vi "alloc_and_project_patterns_dmd.vi"(8 "Path":path, 9 "PicNum":i32, 10 "load patterns":bool, 11 "PictureTime":i32) -> (0 "return array":i32[](array[numeric]), 1 "SeqId":u32, 2 "DevId":u32)   [LabVIEW 2019]
uses:
  <userlib>/alp4395/alp4395.lvlib
  <userlib>/alp4395/alp4395.dll
panel:
  out "path":path
  out "function return 10":i32
  out "function return 6":i32
  out "function return 9":i32
  out "function return 7":i32
  out "function return 5":i32
  out "function return 4":i32
  out "array":u8[][][](array[numeric])
  out "function return 3":i32
  out "function return 2":i32
  out "function return 8":i32
  out "function return":i32
  out "height":i32
  out "width":i32
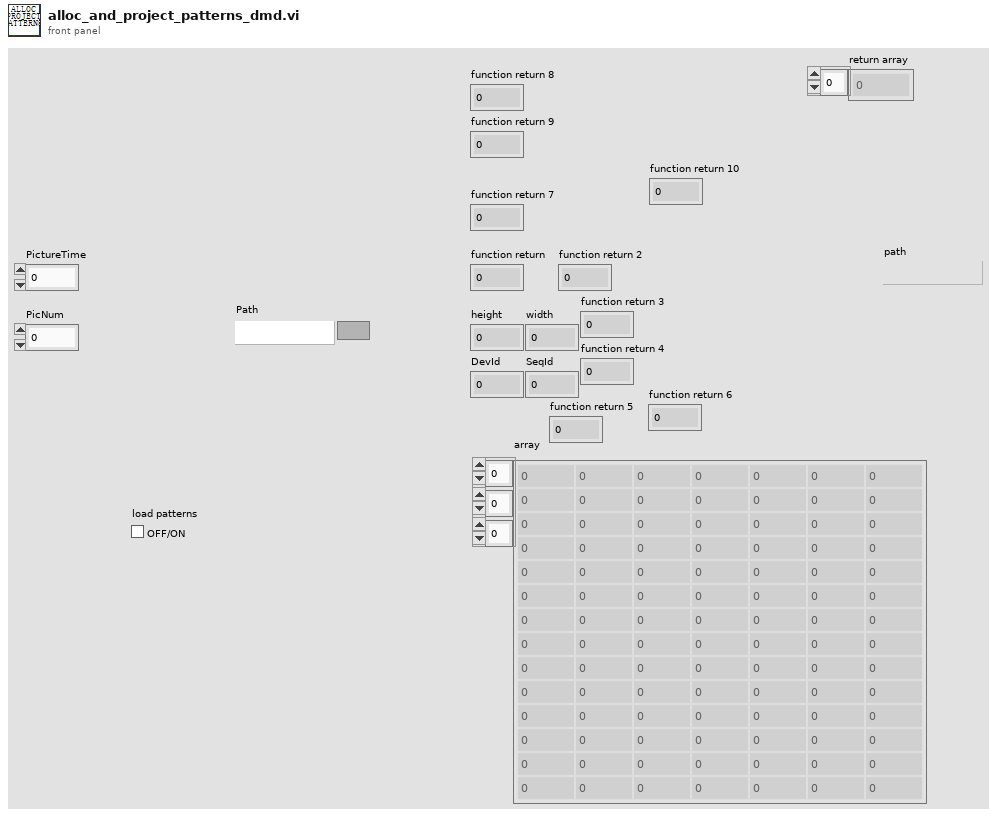
[diagram p1: front panel]
types:
  T1 = typedef "IMAQ Image.ctl" = refnum<image>
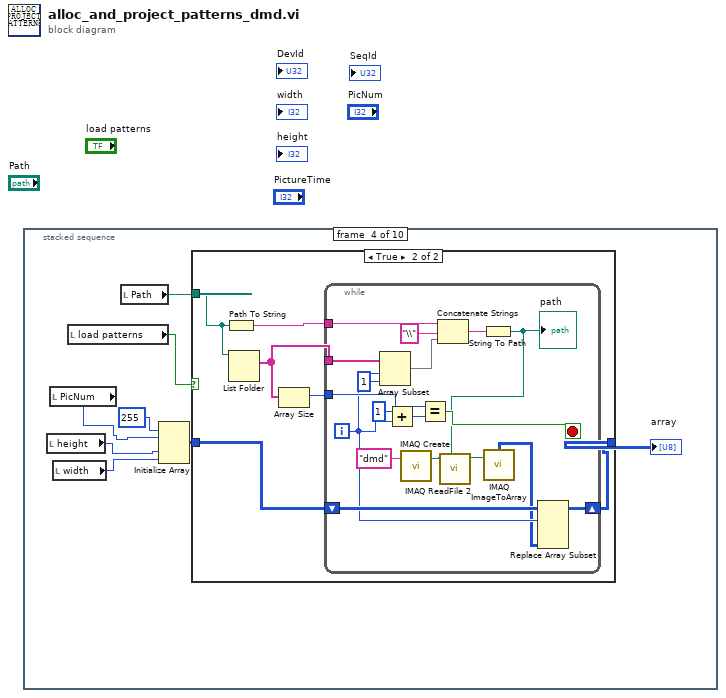
[diagram p0: block diagram]
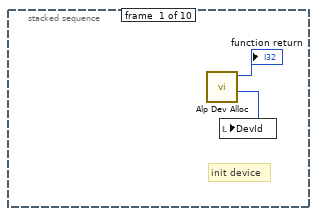
[diagram p2: hidden frame]
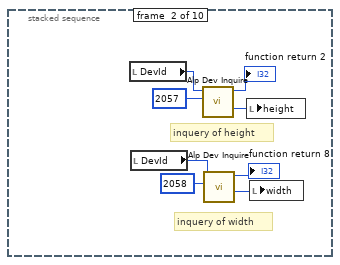
[diagram p3: hidden frame]
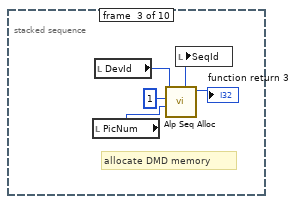
[diagram p4: hidden frame]
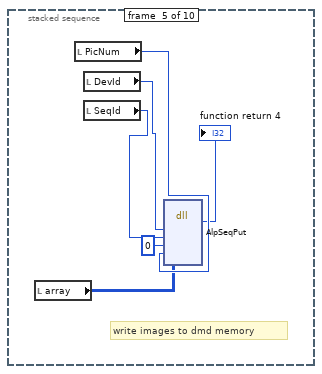
[diagram p6: hidden frame]
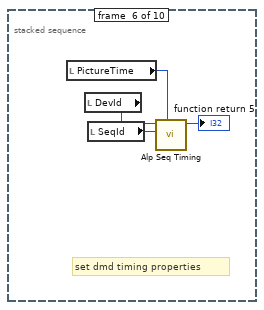
[diagram p7: hidden frame]
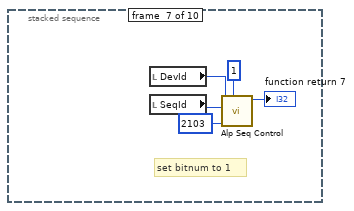
[diagram p8: hidden frame]
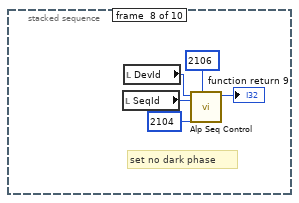
[diagram p9: hidden frame]
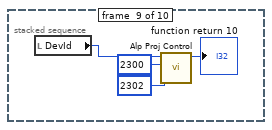
[diagram p10: hidden frame]
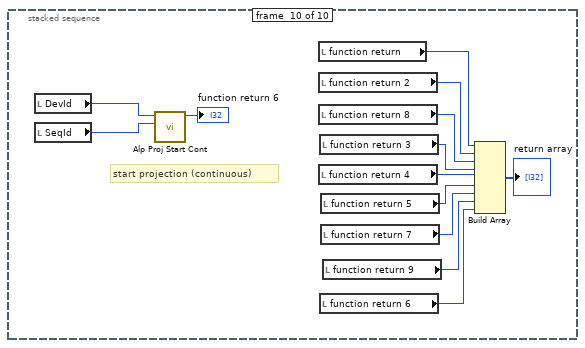
[diagram p11: hidden frame]
diagram:
  n1 = stacked-sequence {
    frame #0 {
      # "init device"
      n2 = call <userlib>:"Alp Dev Alloc.vi"() -> ("DeviceIdPtr out"=w2:u32, "function return"=→"function return":i32)  [unwired: 9 in, 1 out]
      n3 = local write "DevId"(w2) -> ()
    }
    frame #1 {
      # "inquery of width"
      # "inquery of height"
      n4 = local read "DevId"() -> (w8:u32)
      n5 = local read "DevId"() -> (w7:u32)
      n6 = call <userlib>:"Alp Dev Inquire.vi"("InquireType"=2057, "DeviceId"=w8) -> ("UserVarPtr out"=w9:i32, "function return"=→"function return 2":i32)  [unwired: 7 in, 1 out]
      n7 = call <userlib>:"Alp Dev Inquire.vi"("InquireType"=2058, "DeviceId"=w7) -> ("UserVarPtr out"=w5:i32, "function return"=→"function return 8":i32)  [unwired: 7 in, 1 out]
      n8 = local write "height"(w9) -> ()
      n9 = local write "width"(w5) -> ()
    }
    frame #2 {
      # "allocate DMD memory"
      n10 = local read "PicNum"() -> (w12:i32)
      n11 = local read "DevId"() -> (w15:u32)
      n12 = call <userlib>:"Alp Seq Alloc.vi"("PicNum"=w12, "BitPlanes"=1, "DeviceId"=w15) -> ("function return"=→"function return 3":i32, "SequenceIdPtr out"=w14:u32)  [unwired: 6 in, 1 out]
      n13 = local write "SeqId"(w14) -> ()
    }
    frame #3 {
      n14 = local read "height"() -> (w21:i32)
      n15 = local read "PicNum"() -> (w20:i32)
      n16 = local read "width"() -> (w22:i32)
      n17 = local read "load patterns"() -> (w19:bool)
      n18 = local read "Path"() -> (w16:path)
      n19 = Initialize Array(u8 255 ("element"), w20, w21, w22) -> (w18:u8[][][])
      n20 = case shown="True" w19 {
        tunnel: w18 -> [w24 w27]
        tunnel: [w24 w26] -> w17
        tunnel: w16 -> [_ w25]
        frame False {
        }
        frame True {
          n21 = Path To String(path=w25) -> (string=w30:string)
          n22 = List Folder(path=w25) -> (filenames=w29:string[])  [unwired: 3 in, 3 out]
          n23 = Array Size(array=w29) -> (size(s)=w28:i32)
          n24 = while {
            tunnel: w28 -> [w46]
            tunnel: w29 -> [w44]
            tunnel: w30 -> [w42]
            shift-right: [w33] -> w26
            shift-left: w27 -> [w34]
            i -> [w32]
            stop <- w45 stop-if-true
            n25 = Array Subset(array=w44, index=w32, length=1) -> (w40:string[])
            n26 = Add(x=1, y=w32) -> (x+y=w47:i32)
            n27 = call "IMAQ Create"("Image Name"="dmd") -> ("New Image"=w37:T1)  [unwired: 4 in, 1 out]
            n28 = Equal?(x=w46, y=w47) -> (x = y?=w45:bool)
            n29 = Concatenate Strings(w42, "\\", w40) -> (w39:string)
            n30 = String To Path(string=w39) -> (path=w36:path)
            "path" <- w36
            n31 = call "IMAQ ReadFile 2"("File Path"=w36, "Image"=w37) -> ("Image Out"=w35:T1)  [unwired: 5 in, 4 out]
            n32 = call "IMAQ ImageToArray"("Image"=w35) -> ("Image Pixels (U8)"=w31:u8[][])  [unwired: 3 in, 4 out]
            n33 = Replace Array Subset(array=w34, new element=w31, index (dim 0)=w32) -> (w33:u8[][][])  [unwired: 2 in]
          }
        }
      }
      "array" <- w17
    }
    frame #4 {
      # "write images to dmd memory"
      n34 = local read "array"() -> (w50:u8[][][])
      n35 = local read "PicNum"() -> (w52:i32)
      n36 = local read "DevId"() -> (w54:u32)
      n37 = local read "SeqId"() -> (w53:u32)
      n38 = dll-call lib="C:/Program Files/National Instruments/LabVIEW 2019/user.lib/alp4395/alp4395.dll" fn="AlpSeqPut"("DevID"=w54, "SeqID"=w53, "PicOffset"=0, "PicLoad"=w52, "UserArrayPtr"=w50) -> ("return type"=→"function return 4":i32)  [unwired: 3 in, 7 out]
    }
    frame #5 {
      # "set dmd timing properties"
      n39 = local read "PictureTime"() -> (w55:i32)
      n40 = local read "DevId"() -> (w58:u32)
      n41 = local read "SeqId"() -> (w57:u32)
      n42 = call <userlib>:"Alp Seq Timing.vi"("PictureTime"=w55, "SequenceId"=w57, "DeviceId"=w58) -> ("function return"=→"function return 5":i32)  [unwired: 7 in, 1 out]
    }
    frame #6 {
      # "set bitnum to 1"
      n43 = local read "DevId"() -> (w63:u32)
      n44 = local read "SeqId"() -> (w62:u32)
      n45 = call <userlib>:"Alp Seq Control.vi"("ControlValue"=1, "ControlType"=2103, "SequenceId"=w62, "DeviceId"=w63) -> ("function return"=→"function return 7":i32)  [unwired: 6 in, 1 out]
    }
    frame #7 {
      # "set no dark phase"
      n46 = local read "SeqId"() -> (w67:u32)
      n47 = local read "DevId"() -> (w68:u32)
      n48 = call <userlib>:"Alp Seq Control.vi"("ControlValue"=2106, "ControlType"=2104, "SequenceId"=w67, "DeviceId"=w68) -> ("function return"=→"function return 9":i32)  [unwired: 6 in, 1 out]
    }
    frame #8 {
      n49 = local read "DevId"() -> (w72:u32)
      n50 = call <userlib>:"Alp Proj Control.vi"("ControlValue"=2302, "ControlType"=2300, "DeviceId"=w72) -> ("function return"=→"function return 10":i32)  [unwired: 7 in, 1 out]
    }
    frame #9 {
      # "start projection (continuous)"
      n51 = local read "DevId"() -> (w85:u32)
      n52 = local read "SeqId"() -> (w84:u32)
      n53 = call <userlib>:"Alp Proj Start Cont.vi"("SequenceId"=w84, "DeviceId"=w85) -> ("function return"=→"function return 6":i32)  [unwired: 8 in, 1 out]
      n54 = local read "function return"() -> (w73:i32)
      n55 = local read "function return 2"() -> (w74:i32)
      n56 = local read "function return 8"() -> (w75:i32)
      n57 = local read "function return 4"() -> (w77:i32)
      n58 = local read "function return 3"() -> (w76:i32)
      n59 = local read "function return 6"() -> (w81:i32)
      n60 = local read "function return 5"() -> (w78:i32)
      n61 = local read "function return 7"() -> (w79:i32)
      n62 = local read "function return 9"() -> (w80:i32)
      n63 = Build Array(w73, w74, w75, w76, w77, w78, w79, w80, w81) -> (→"return array":i32[])
    }
  }
